vi "ScanFeedback.vi"(2 "measurement type":T1(tab)) -> (1 "V breakdown":dbl, 5 "V depletion":dbl, 6 "Maximum current fluctuations [%]":dbl[](array[numeric]), 8 "Ris [MOhm]":dbl, 9 "Cis @300V [pF/cm]":dbl)   [LabVIEW 2018]
uses:
  globals/QC_RunInformation.vi
  <vilib>/Analysis/NI_AALPro.lvlib
  <vilib>/Analysis/NI_AALBase.lvlib
panel:
  out "MEAN":dbl
  out "STD":dbl
  out "Index lin fit 1":dbl
  out "Slope":dbl
  out "capSquare1":dbl[](array[numeric])
  out "volts1":dbl[](array[numeric])
  out "volts2":dbl[](array[numeric])
  out "capSquare2":dbl[](array[numeric])
  out "deriv":dbl[](array[numeric])
  out "Slope 2":dbl
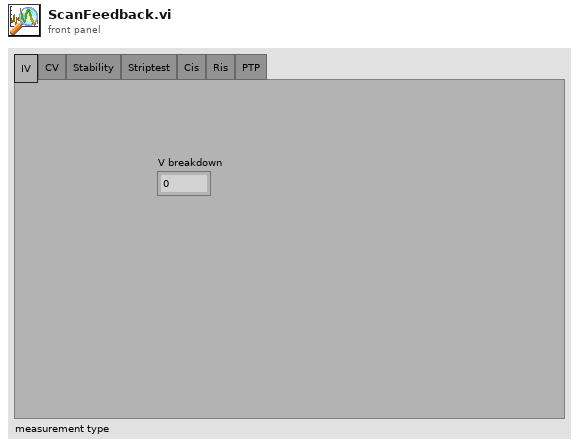
[diagram p1: front panel]
types:
  T1 = enum32{"IV", "CV", "Stability", "Striptest", "Cis", "Ris", "PTP"}
  T2 = cluster{"Sensor Serial No.:":string, "Wafer:":string, "Batch:":string, "Manufacturer:":string, "Device Category:":string, "Database Serial No.:":string, "Date Initiated:":string, "Time Initiated:":string, "Test":string, "Probeplan used:":string, "End of Run Status":dbl, "End of Run comment:":string, "User:":string, "Vbias SMU":string, "LCR":string, "Test SMU":string, "Test DMM":string, "Comments":string, "Measurement results":cluster{"IV":string, "CV":string, "Cis":string, "Ris":string, "Stability":string, "PTP":string, "Striptest":string}}
  T3 = enum16{"Reset", "Read Array", "Read Element", "Write Element", "Write Array", "Add Element", "Add Array"}
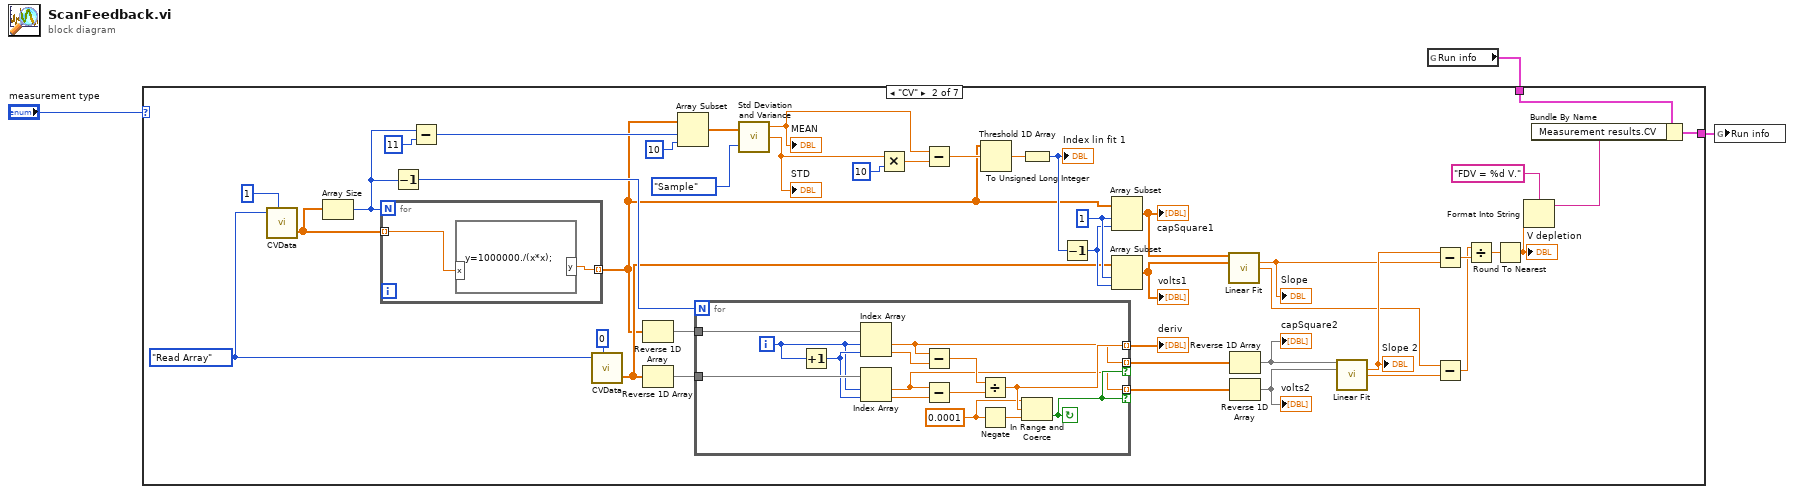
[diagram p0: block diagram]
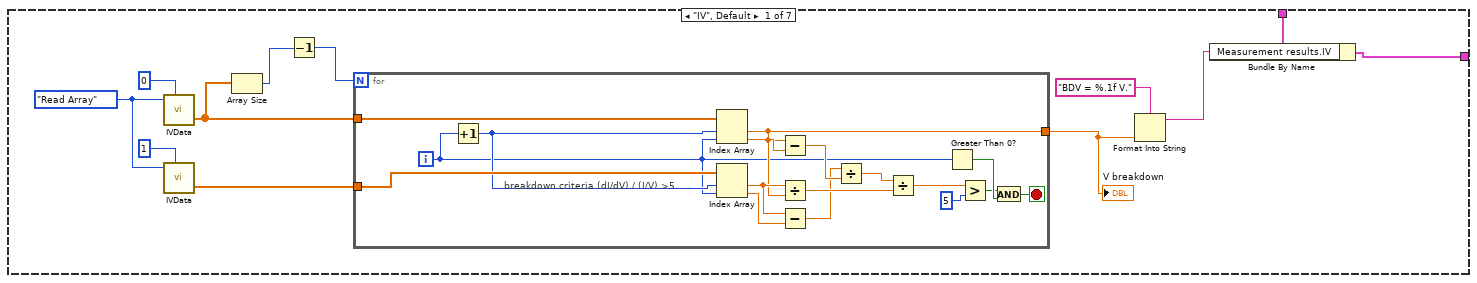
[diagram p2: hidden frame]
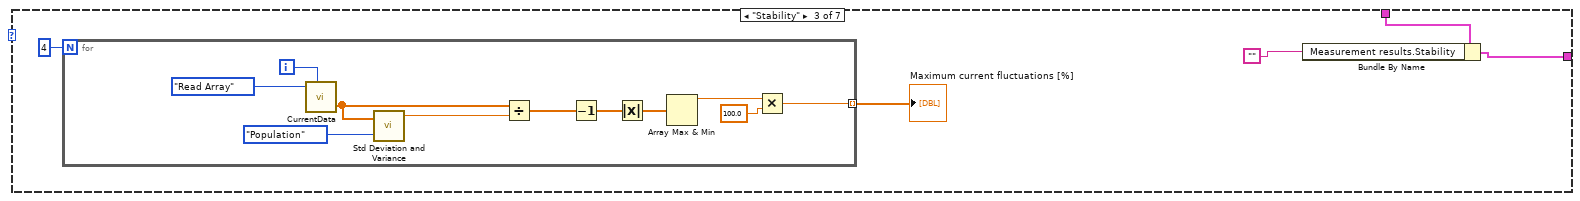
[diagram p3: hidden frame]
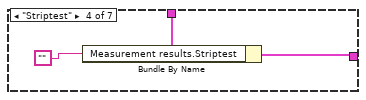
[diagram p4: hidden frame]
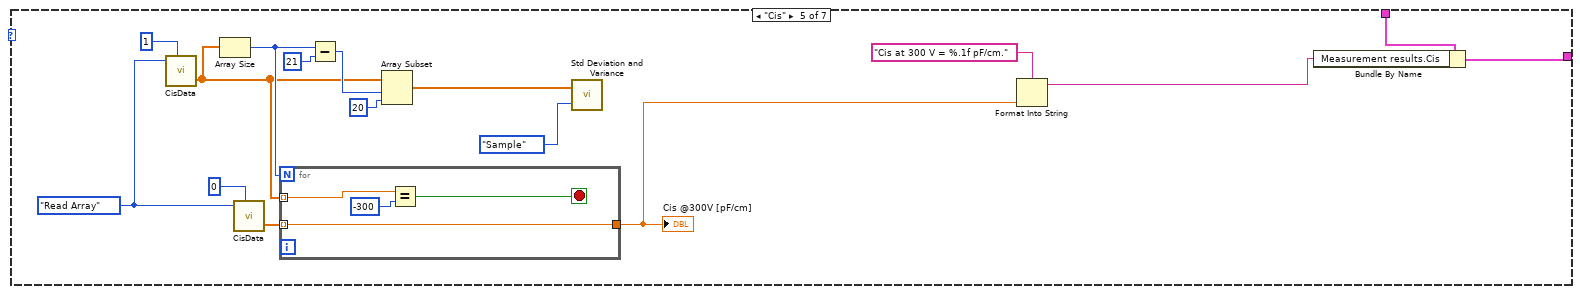
[diagram p5: hidden frame]
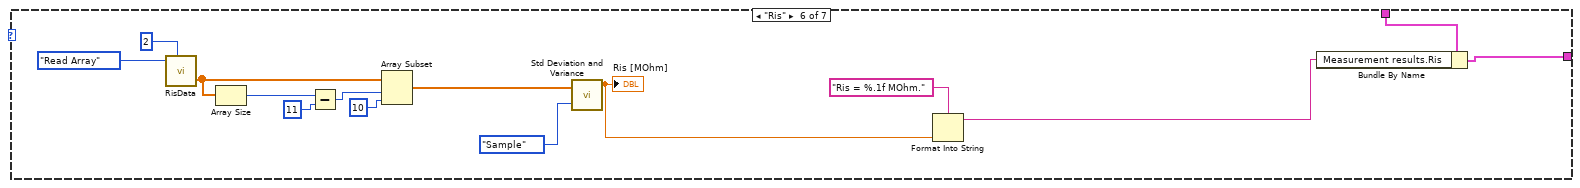
[diagram p6: hidden frame]
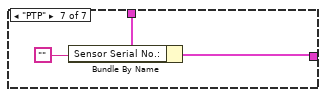
[diagram p7: hidden frame]
diagram:
  n1 = global read "QC_RunInformation.vi" "Run info"() -> (w2:T2)
  n2 = case shown="\"CV\"" "measurement type" {
    tunnel: w2 -> [w8 w35 w94 w110 w113 w133 w147]
    tunnel: [w6 w33 w92 w108 w111 w131 w145] -> w1
    frame "IV", Default {
      w13 = T3."Read Array" ("Action")
      n3 = call "IVData.vi"("Action"=w13, "Array No."=0) -> ("Array OUT"=w5:dbl[])  [unwired: 3 in, 1 out]
      n4 = call "IVData.vi"("Action"=w13, "Array No."=1) -> ("Array OUT"=w12:dbl[])  [unwired: 3 in, 1 out]
      n5 = Array Size(array=w5) -> (size(s)=w4:i32)
      n6 = Decrement(x=w4) -> (x-1=w11:i32)
      n7 = for {
        N: w11 -> [_]
        tunnel: w5 -> [w31]
        tunnel: w12 -> [w32]
        tunnel: [w20] -> w9
        i -> [w18]
        stop <- w16 stop-if-true
        # "breakdown criteria (dI/dV) / (I/V) >5"
        n8 = Increment(x=w18) -> (x+1=w28:i32)
        n9 = Index Array(array=w31, index #1=w28, index #2=w18) -> (element #1=w20:dbl, element #2=w30:dbl)
        n10 = Index Array(array=w32, index #1=w28, index #2=w18) -> (element #1=w23:dbl, element #2=w29:dbl)
        n11 = Subtract(x=w20, y=w30) -> (x-y=w25:dbl)
        n12 = Divide(x=w23, y=w20) -> (x/y=w26:dbl)
        n13 = Subtract(x=w23, y=w29) -> (x-y=w24:dbl)
        n14 = Divide(x=w24, y=w25) -> (x/y=w27:dbl)
        n15 = Divide(x=w27, y=w26) -> (x/y=w21:dbl)
        n16 = Greater Than 0?(x=w18) -> (x > 0?=w19:bool)
        n17 = Greater?(x=w21, y=5) -> (0:w17:bool)
        n18 = And(x=w17, y=w19) -> (x .and. y?=w16:bool)
      }
      "V breakdown" <- w9
      n19 = Format Into String(format string="BDV = %.1f V.", w9) -> (resulting string=w7:string)  [unwired: 2 in, 1 out]
      n20 = Bundle By Name(cluster=w8, "Measurement results.IV"=w7) -> (w6:T2)
    }
    frame "CV" {
      w48 = T3."Read Array" ("Action")
      w45 = 1
      n21 = call "CVData.vi"("Action"=w48, "Array No."=1) -> ("Array OUT"=w39:dbl[])  [unwired: 3 in, 1 out]
      n22 = Array Size(array=w39) -> (size(s)=w40:i32)
      n23 = for {
        N: w40 -> [_]
        tunnel: w39 -> [w77] mode=indexing
        tunnel: [w76] -> w38 mode=indexing
        n24 = formula code="y=1000000./(x*x);"("x"=w77) -> ("y"=w76:dbl)
      }
      n25 = Decrement(x=w40) -> (x-1=w60:i32)
      n26 = Subtract(x=w40, y=11) -> (x-y=w74:i32)
      n27 = call "CVData.vi"("Action"=w48, "Array No."=0) -> ("Array OUT"=w42:dbl[])  [unwired: 3 in, 1 out]
      n28 = Reverse 1D Array(array=w38) -> (reversed array=w63:dbl[])
      n29 = Reverse 1D Array(array=w42) -> (reversed array=w41:dbl[])
      n30 = Array Subset(array=w38, index=w74, length=10) -> (w72:dbl[])
      n31 = for {
        N: w60 -> [_]
        tunnel: w63 -> [w91]
        tunnel: [w84] -> w62 mode=indexing if=w85
        tunnel: [w80] -> w59 mode=indexing if=w85
        tunnel: [w88] -> w56 mode=indexing
        tunnel: w41 -> [w83]
        i -> [w81]
        stop <- w85 continue-if-true
        w86 = 0.0001
        n32 = Increment(x=w81) -> (x+1=w82:i32)
        n33 = Index Array(array=w91, index #1=w81, index #2=w82) -> (element #1=w84:dbl, element #2=w89:dbl)
        n34 = Index Array(array=w83, index #1=w81, index #2=w82) -> (element #1=w80:dbl, element #2=w79:dbl)
        n35 = Subtract(x=w84, y=w89) -> (x-y=w90:dbl)
        n36 = Subtract(x=w80, y=w79) -> (x-y=w78:dbl)
        n37 = Divide(x=w90, y=w78) -> (x/y=w88:dbl)
        n38 = Negate(x=w86) -> (-x=w87:dbl)
        n39 = In Range and Coerce(upper limit=w86, x=w88, lower limit=w87) -> (In Range?=w85:bool)  [unwired: 1 out]
      }
      "deriv" <- w56
      n40 = call <vilib>:"Std Deviation and Variance.vi"("X"=w72, "Weighting (Sample)"=enum16{"Sample", "Population"}."Sample") -> ("mean"=w68:dbl, "standard deviation"=w57:dbl)  [unwired: 1 out]
      "MEAN" <- w68
      "STD" <- w57
      n41 = Multiply(x=w57, y=10) -> (x*y=w69:dbl)
      n42 = Subtract(x=w68, y=w69) -> (x-y=w67:dbl)
      n43 = Threshold 1D Array(2:w67, 3:w38) -> (0:w66:dbl)  [unwired: 1 in]
      n44 = To Unsigned Long Integer(number=w66) -> (unsigned 32bit integer=w65:u32)
      "Index lin fit 1" <- w65
      n45 = Decrement(x=w65) -> (x-1=w44:u32)
      n46 = Array Subset(array=w38, index=w45, length=w44) -> (w64:dbl[])
      "capSquare1" <- w64
      n47 = Array Subset(array=w42, index=w45, length=w44) -> (w43:dbl[])
      "volts1" <- w43
      n48 = call <vilib>:"Linear Fit.vi"("Y"=w64, "X"=w43) -> ("slope"=w54:dbl, "intercept"=w52:dbl)  [unwired: 9 in, 3 out]
      "Slope" <- w54
      n49 = Reverse 1D Array(array=w62) -> (reversed array=w61:dbl[])
      "capSquare2" <- w61
      n50 = Reverse 1D Array(array=w59) -> (reversed array=w58:dbl[])
      "volts2" <- w58
      n51 = call <vilib>:"Linear Fit.vi"("Y"=w61, "X"=w58) -> ("slope"=w55:dbl, "intercept"=w53:dbl)  [unwired: 9 in, 3 out]
      "Slope 2" <- w55
      n52 = Subtract(x=w55, y=w54) -> (x-y=w51:dbl)
      n53 = Subtract(x=w52, y=w53) -> (x-y=w50:dbl)
      n54 = Divide(x=w50, y=w51) -> (x/y=w49:dbl)
      n55 = Round To Nearest(number=w49) -> (nearest integer value=w37:dbl)
      "V depletion" <- w37
      n56 = Format Into String(format string="FDV = %d V.", w37) -> (resulting string=w34:string)  [unwired: 2 in, 1 out]
      n57 = Bundle By Name(cluster=w35, "Measurement results.CV"=w34) -> (w33:T2)
    }
    frame "Stability" {
      n58 = for {
        N: 4 -> [_]
        tunnel: [w97] -> w95 mode=indexing
        i -> [w106]
        n59 = call "CurrentData.vi"("Action"=T3."Read Array", "Array No."=w106) -> ("Array OUT"=w103:dbl[])  [unwired: 3 in, 1 out]
        n60 = call <vilib>:"Std Deviation and Variance.vi"("X"=w103, "Weighting (Sample)"=enum16{"Sample", "Population"}."Population") -> ("mean"=w104:dbl)  [unwired: 2 out]
        n61 = Divide(x=w103, y=w104) -> (x/y=w102:dbl[])
        n62 = Decrement(x=w102) -> (x-1=w101:dbl[])
        n63 = Absolute Value(x=w101) -> (abs(x)=w100:dbl[])
        n64 = Array Max & Min(array=w100) -> (max value=w99:dbl)  [unwired: 3 out]
        n65 = Multiply(x=w99, y=100.0) -> (x*y=w97:dbl)
      }
      "Maximum current fluctuations [%]" <- w95
      n66 = Bundle By Name(cluster=w94, "Measurement results.Stability"="") -> (w92:T2)
    }
    frame "Striptest" {
      n67 = Bundle By Name(cluster=w110, "Measurement results.Striptest"="") -> (w108:T2)
    }
    frame "Cis" {
      w120 = T3."Read Array" ("Action")
      n68 = call "CisData.vi"("Action"=w120, "Array No."=1) -> ("Array OUT"=w117:dbl[])  [unwired: 3 in, 1 out]
      n69 = Array Size(array=w117) -> (size(s)=w118:i32)
      n70 = call "CisData.vi"("Action"=w120, "Array No."=0) -> ("Array OUT"=w116:dbl[])  [unwired: 3 in, 1 out]
      n71 = for {
        N: w118 -> [_]
        tunnel: w117 -> [w129] mode=indexing
        tunnel: w116 -> [w127] mode=indexing
        tunnel: [w127] -> w114
        stop <- w128 stop-if-true
        n72 = Equal?(x=w129, y=-300) -> (x = y?=w128:bool)
      }
      "Cis @300V [pF/cm]" <- w114
      n73 = Subtract(x=w118, y=21) -> (x-y=w122:i32)
      n74 = Array Subset(array=w117, index=w122, length=20) -> (w121:dbl[])
      n75 = call <vilib>:"Std Deviation and Variance.vi"("X"=w121, "Weighting (Sample)"=enum16{"Sample", "Population"}."Sample") -> ()  [unwired: 3 out]
      n76 = Format Into String(format string="Cis at 300 V = %.1f pF/cm.", w114) -> (resulting string=w112:string)  [unwired: 2 in, 1 out]
      n77 = Bundle By Name(cluster=w113, "Measurement results.Cis"=w112) -> (w111:T2)
    }
    frame "Ris" {
      n78 = call "RisData.vi"("Action"=T3."Read Array", "Array No."=2) -> ("Array OUT"=w136:dbl[])  [unwired: 3 in, 1 out]
      n79 = Array Size(array=w136) -> (size(s)=w143:i32)
      n80 = Subtract(x=w143, y=11) -> (x-y=w140:i32)
      n81 = Array Subset(array=w136, index=w140, length=10) -> (w139:dbl[])
      n82 = call <vilib>:"Std Deviation and Variance.vi"("X"=w139, "Weighting (Sample)"=enum16{"Sample", "Population"}."Sample") -> ("mean"=w134:dbl)  [unwired: 2 out]
      "Ris [MOhm]" <- w134
      n83 = Format Into String(format string="Ris = %.1f MOhm.", w134) -> (resulting string=w132:string)  [unwired: 2 in, 1 out]
      n84 = Bundle By Name(cluster=w133, "Measurement results.Ris"=w132) -> (w131:T2)
    }
    frame "PTP" {
      n85 = Bundle By Name(cluster=w147, "Sensor Serial No.:"="") -> (w145:T2)
    }
  }
  n86 = global write "QC_RunInformation.vi" "Run info"(w1) -> ()
